vi "Encode I32.vi"(9 "Pixel Offset (0)":i32, 10 "I32":i32, 11 "Image In":u8[](array[numeric])) -> (3 "Image Out":u8[](array[numeric]))   [LabVIEW 2020]
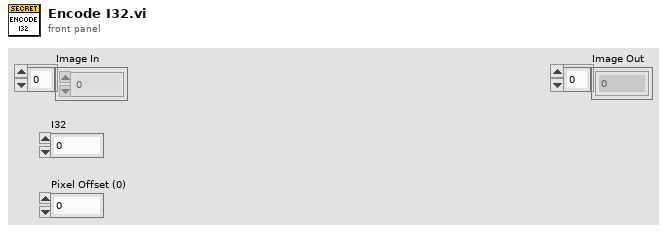
[diagram p1: front panel]
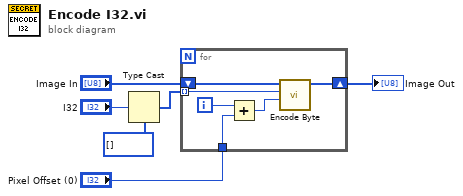
[diagram p0: block diagram]
diagram:
  n1 = Type Cast(type=u8[] [] ("Compressed Message 2"), x="I32") -> (*(type *) &x=w5:u8[])
  n2 = for {
    tunnel: w5 -> [w12] mode=indexing
    shift-right: [w10] -> w3
    shift-left: "Image In" -> [w11]
    tunnel: "Pixel Offset (0)" -> [w7]
    i -> [w9]
    n3 = Add(x=w9, y=w7) -> (x+y=w8:i32)
    n4 = call "Encode Byte.vi"("Pixel Offset"=w8, "Byte To Encode"=w12, "Image In"=w11) -> ("Image Out"=w10:u8[])  [unwired: 8 in]
  }
  "Image Out" <- w3
